vi "test_LocationFGV_ReresolveLocationErrors_LocationNotResolved.vi"(8 "error in":errorcluster) -> (0 "error out":errorcluster, 2 "result":string, 3 "pass":bool)   [LabVIEW 2020, in "MeasurementServerTests.lvlib" / "Discovery Tests.lvlib"]
uses:
  Discovery Tests.lvlib
  Fake Service Location Generator Action.ctl
  Runtime/Measurements/Measurement Plugin Discovery V1/TypeDefs/Service Location FGV Action.ctl
  Runtime/Measurements/Measurement Plugin Discovery V1/Measurement Plugin Discovery V1.lvlib
  Runtime/Generated/Measurement Plugin Discovery Client/RPC Messages/ni_measurementlink_discovery_v1_ResolveServiceRequest.ctl
  Runtime/Generated/Measurement Plugin Discovery Client/Measurement Plugin Discovery Client.lvlib
  MeasurementServerTests.lvlib
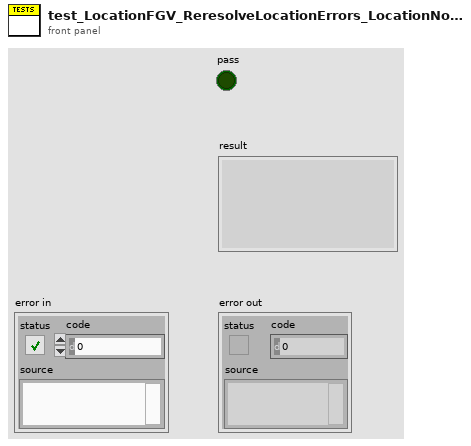
[diagram p1: front panel]
types:
  T1 = typedef "MeasurementServerTests.lvlib/Discovery Tests.lvlib/Fake Service Location Generator Action.ctl" = enum16{"Generate New Location", "Reset", "Error on Next Call"}
  T2 = typedef "Measurement Plugin Discovery Client.lvlib/ni_measurementlink_discovery_v1_ResolveServiceRequest.ctl" = cluster{"provided_interface":string, "service_class":string}
  T3 = typedef "Measurement Plugin Discovery V1.lvlib/Service Location FGV Action.ctl" = enum16{"Get Service Location", "Reresolve Service Location"}
  T4 = typedef "Measurement Plugin Discovery Client.lvlib/ni_measurementlink_discovery_v1_ServiceLocation.ctl" = cluster{"location":string, "insecure_port":string, "ssl_authenticated_port":string}
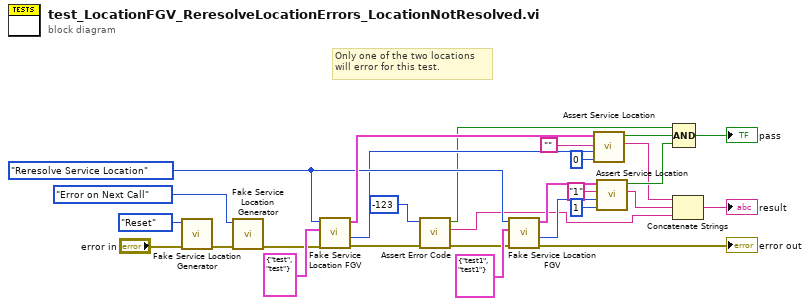
[diagram p0: block diagram]
diagram:
  w22 = Service_Location_FGV_Action."Reresolve Service Location" ("action")
  # "Only one of the two locations\nwill error for this test."
  n1 = call "Fake Service Location Generator.vi"("error in"="error in", "action"=Fake_Service_Location_Generator_Action."Reset") -> ("error out"=w9:errorcluster)  [unwired: 8 in, 1 out]
  n2 = call "Fake Service Location Generator.vi"("error in"=w9, "action"=Fake_Service_Location_Generator_Action."Error on Next Call") -> ("error out"=w7:errorcluster)  [unwired: 8 in, 1 out]
  n3 = call "Fake Service Location FGV.vi"("error in"=w7, "resolve service request"=T2 {"provided_interface"="test", "service_class"="test"}, "action"=w22) -> ("error out"=w5:errorcluster, "unique id out"=w21:u64, "service location"=w26:T4)  [unwired: 6 in]
  n4 = call "Assert Error Code.vi"("error in"=w5, "expected error code"=-123) -> ("error out"=w4:errorcluster, "details"=w1:string, "error code match?"=w2:bool)  [unwired: 7 in]
  n5 = call "Fake Service Location FGV.vi"("error in"=w4, "resolve service request"=T2 {"provided_interface"="test1", "service_class"="test1"}, "action"=w22) -> ("error out"=→"error out":errorcluster, "unique id out"=w17:u64, "service location"=w19:T4)  [unwired: 6 in]
  n6 = call "Assert Service Location.vi"("expected unique id"=u64 0, "actual unique id"=w21, "expected service location port"="", "actual service location"=w26) -> ("result"=w12:string, "pass"=w14:bool)  [unwired: 6 in]
  n7 = call "Assert Service Location.vi"("expected unique id"=u64 1, "actual unique id"=w17, "expected service location port"="1", "actual service location"=w19) -> ("result"=w10:string, "pass"=w15:bool)  [unwired: 6 in]
  n8 = Compound Arithmetic op=AND(w2, w14, w15) -> (→"pass":bool)
  n9 = Concatenate Strings(w12, w10, w1) -> (→"result":string)
